vi "Convert String to Bits Array.vi"(11 "I_String":string) -> (3 "O_Bits Array":i16[](array[numeric]))   [LabVIEW 2015]
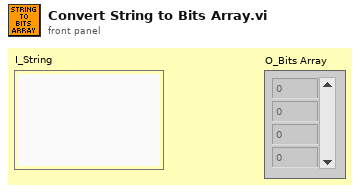
[diagram p1: front panel]
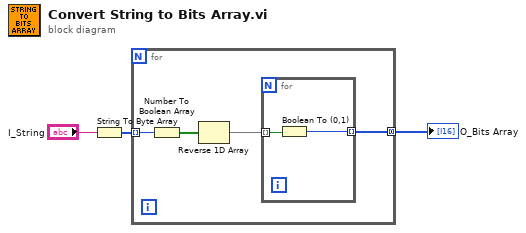
[diagram p0: block diagram]
diagram:
  n1 = String To Byte Array(string="I_String") -> (unsigned byte array=w2:u8[])
  n2 = for {
    tunnel: w2 -> [w7] mode=indexing
    tunnel: [w5] -> w1 mode=concatenating
    n3 = Number To Boolean Array(number=w7) -> (Boolean array=w6:bool[])
    n4 = Reverse 1D Array(array=w6) -> (reversed array=w4:bool[])
    n5 = for {
      tunnel: w4 -> [w9] mode=indexing
      tunnel: [w8] -> w5 mode=indexing
      n6 = Boolean To (0,1)(Boolean=w9) -> (0, 1=w8:i16)
    }
  }
  "O_Bits Array" <- w1
